vi "CANopen SYNC.vi"() -> ()   [LabVIEW 2016]
doc: "This example demonstrates how to send CANopen SYNC message to the network."
uses:
  <vilib>/userdefined/High Color/nirio_resource_hc.ctl
  <vilib>/Platform/TimedLoop/XDataNode/timing_clust.ctl
  <vilib>/Platform/TimedLoop/XDataNode/nitl_modes.ctl
  <vilib>/Platform/TimedLoop/XDataNode/wakeup.ctl
  <vilib>/FPGAPlugInAG/cRIO-9033/niLvFpga_Open_cRIO-9033.vi
  <vilib>/rvi/interface/common/dynamic/niFpgaDynamicAddResources.vi
  <vilib>/CANopenLib/CANOPEN.llb/CANopen Interface Create.vi
  <vilib>/CANopenLib/CANOPEN.llb/CANopen SYNC Create.vi
  <vilib>/CANopenLib/CANOPEN.llb/CANopen SYNC Start.vi
  <vilib>/CANopenLib/CANOPEN.llb/CANopen SYNC Close.vi
  <vilib>/CANopenLib/CANOPEN.llb/CANopen Interface Close.vi
  <vilib>/FPGAPlugInAG/Dynamic/niLvFpga_Close_Dynamic.vi
  <vilib>/rvi/interface/nirviOpenFPGA/nirviOpenFPGA.xnode
  Users/s163601/Desktop/05-28/FPGA Bitfiles/project_FPGATarget_MainFPGA_S9ZLErdeBuw.lvbitx
  Users/s163601/Desktop/05-28/RT/FPGA/MainFPGA.vi
  <vilib>/Platform/TimedLoop/XDataNode/XDataNode.xnode
  <vilib>/rvi/interface/nirviCloseFPGA/nirviCloseFPGA.xnode
  <vilib>/Platform/TimedLoop/XDataNode/XDNodeRunTimeDep.lvlib
panel:
  in  "error in":errorcluster
  in  "stop":bool
  in  "period (ms)":i64=10
  in  "counter overflow value":u8=5
  in  "node-ID":u8=1 min=1 max=127 step=1
  in  "baud rate":u32(ring)=2 items=["1 Mbit/s"=0, "800 kbit/s"=1, "500 kbit/s"=2, "250 kbit/s"=3, "125 kbit/s"=4, "50 kbit/s"=6, "20 kbit/s"=7, "10 kbit/s"=8]
  in  "CANopen interface":u32(ring) items=["CANopen01", "CANopen02", "CANopen03", "CANopen04", "CANopen05", "CANopen06", "CANopen07", "CANopen08", "CANopen09", "CANopen10", "CANopen11", "CANopen12", "CANopen13", "CANopen14", "CANopen15", "CANopen16", "CANopen17", "CANopen18", "CANopen19", "CANopen20", "CANopen21", "CANopen22", "CANopen23", "CANopen24", "CANopen25", "CANopen26", "CANopen27", "CANopen28", "CANopen29", "CANopen30", "CANopen31", "CANopen32"]
  # "Overview: This example demonstrates how to send CANopen SYNC message to the network.\nRequirements: Connect CANopen module with a slave device. \nInstructions:\n1. Specify the values of CANopen interface, baud rate of the CANopen interface, node-ID of the slave device and \n    counter overflow value of the the SYNC object.\n2. Run this VI.\n3. Click STOP to stop the VI."
  # "Create CANopen interface and SYNC object"
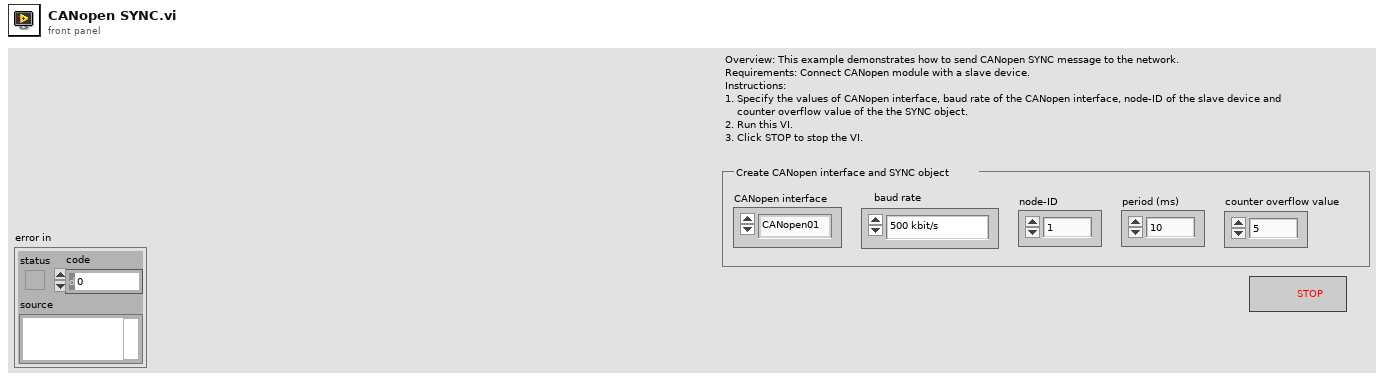
[diagram p1: front panel]
types:
  T1 = typedef "nirio_resource_hc.ctl" = tag
  T2 = typedef "XDNodeRunTimeDep.lvlib/timing_clust.ctl" = cluster{"Expected End [f-1]":u64, "Actual End [f-1]":u64, "Finished Late? [f-1]":bool, "Expected End [i-1]":u64, "Actual End [i-1]":u64, "Finished Late? [i-1]":bool, "Expected Start [i]":u64, "Actual Start [i]":u64, "Expected Start [f]":u64, "Actual Start [f]":u64, "Source Name":string, "Structure Name":string, "Period":i64, "Deadline":i64, "Offset":i64, "Start":i64, "Priority":i32, "Timeout":i32, "Mode":T3, "Wakeup Reason":T4, "Error":errorcluster, "Source Type":string, "Secondary Source Type":string, "Global End Time":u64, "Global Start Time":u64, "Frame Duration":u64, "Iteration Duration":u64, "Assigned CPU":i32, "I/O Scan Engine Mode":u32}
  T3 = typedef "XDNodeRunTimeDep.lvlib/nitl_modes.ctl" = enum32{"No Change", "Process missed periods, maintain original phase", "Discard missed periods, maintain original phase", "Process missed periods, ignore original phase", "Discard missed periods, ignore original phase"}
  T4 = typedef "XDNodeRunTimeDep.lvlib/wakeup.ctl" = enum32{"Normal", "Aborted", "Asynchronous wakeup", "Timing source error", "Timed loop error", "Timeout"}
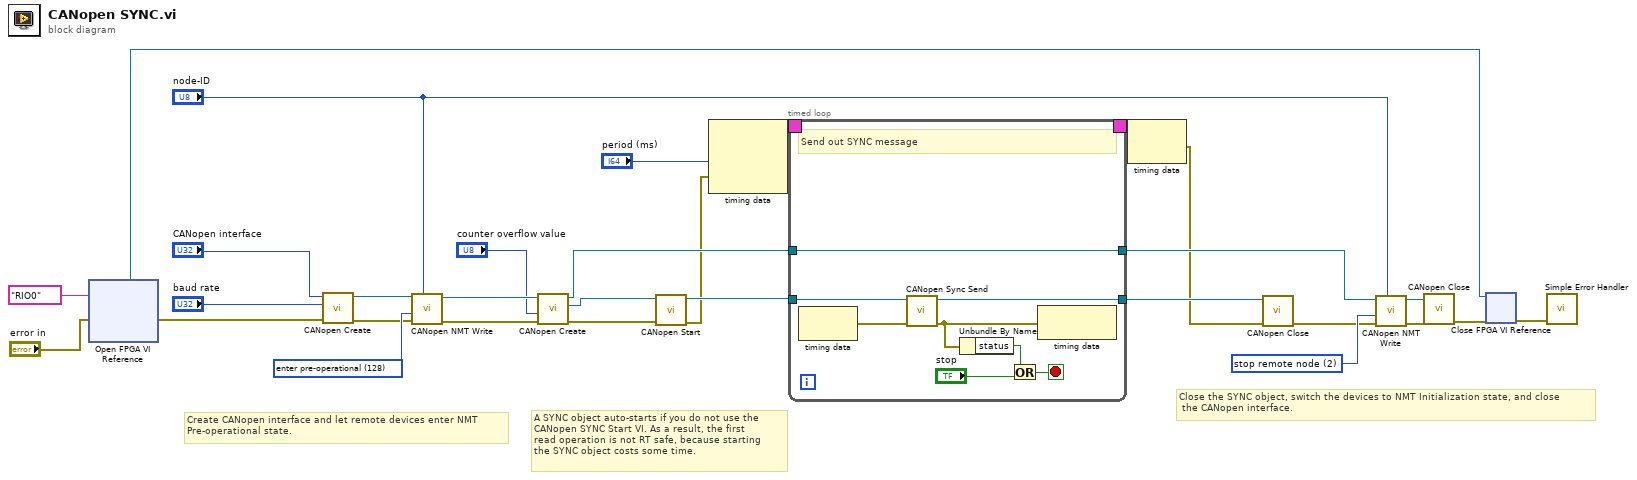
[diagram p0: block diagram]
diagram:
  w16 = u16 2 items=["start remote node"=1, "stop remote node"=2, "enter pre-operational"=128, "reset node"=129, "reset communication"=130] ("command")
  w26 = u16 128 items=["start remote node"=1, "stop remote node"=2, "enter pre-operational"=128, "reset node"=129, "reset communication"=130] ("command")
  # "A SYNC object auto-starts if you do not use the \nCANopen SYNC Start VI. As a result, the first \nread operation is not RT safe, because starting \nthe SYNC object costs some time."
  # "Close the SYNC object, switch the devices to NMT Initialization state, and close\n the CANopen interface."
  # "Create CANopen interface and let remote devices enter NMT\nPre-operational state."
  n1 = xnode ("Open FPGA VI Reference")("error in"="error in", "resource name"=T1 "RIO0") -> ("FPGA VI Reference Out"=w1:refnum<k20>, "error out"=w4:errorcluster)
  n2 = call-poly <vilib>:"CANopen Create.vi"("error in (no error)"=w4, "baud rate"="baud rate", "interface name"="CANopen interface") -> ("error out"=w8:errorcluster, "interface object out"=w25:refnum<k20>)  [unwired: 7 in]
  n3 = call <vilib>:"CANopen NMT Write.vi"("node-ID (0)"="node-ID", "error in (no error)"=w8, "command"=w26, "interface object in"=w25) -> ("error out"=w24:errorcluster, "interface object out"=w23:refnum<k20>)  [unwired: 6 in]
  n4 = call-poly <vilib>:"CANopen Create.vi"("error in (no error)"=w24, "counter overflow value (0)"="counter overflow value", "interface object in"=w23) -> ("error out"=w7:errorcluster, "SYNC object out"=w13:refnum<k20>, "interface object out"=w20:refnum<k20>)  [unwired: 6 in]
  n5 = call-poly <vilib>:"CANopen Start.vi"("error in (no error)"=w7, "SYNC object in"=w13) -> ("error out"=w11:errorcluster, "SYNC object out"=w19:refnum<k20>)  [unwired: 8 in]
  n6 = node-c288("period (ms)", w11) -> (w30:T2)  [unwired: 1 in]
  n7 = timed-loop {
    tunnel: w19 -> [w38]
    tunnel: [w37] -> w21
    tunnel: [w36] -> w14
    tunnel: w20 -> [w36]
    timing: w30 -> [_]
    timing-out: [_] -> w29
    stop <- w35 stop-if-true
    # "Send out SYNC message"
    n8 = node-c288() -> (w32:errorcluster)  [unwired: 1 in]
    n9 = call <vilib>:"CANopen Sync Send.vi"("error in (no error)"=w32, "SYNC object in"=w38) -> ("error out"=w31:errorcluster, "SYNC object out"=w37:refnum<k20>)  [unwired: 8 in]
    n10 = Unbundle By Name(w31) -> ("status"=w33:bool)
    n11 = Or(x=w33, y="stop") -> (x .or. y?=w35:bool)
    n12 = node-c288(w31) -> ()  [unwired: 1 out]
  }
  n13 = node-c288(w29) -> (w9:errorcluster)
  n14 = call-poly <vilib>:"CANopen Close.vi"("error in (no error)"=w9, "SYNC object in"=w21) -> ("error out"=w15:errorcluster)  [unwired: 9 in]
  n15 = call <vilib>:"CANopen NMT Write.vi"("node-ID (0)"="node-ID", "error in (no error)"=w15, "command"=w16, "interface object in"=w14) -> ("error out"=w18:errorcluster, "interface object out"=w17:refnum<k20>)  [unwired: 6 in]
  n16 = call-poly <vilib>:"CANopen Close.vi"("error in (no error)"=w18, "interface object in"=w17) -> ("error out"=w3:errorcluster)  [unwired: 9 in]
  n17 = xnode "Close FPGA VI Reference"("FPGA VI Reference In"=w1, "error in"=w3) -> ("error out"=w2:errorcluster)
  n18 = call <vilib>:"Simple Error Handler.vi"("error in (no error)"=w2) -> ()  [unwired: 4 in, 5 out]
